vi "Simulation Configuration from Command-Line.vi"(8 "error in":errorcluster, 11 "simulation configuration in":T1={"maxTime"=5.0, "enableVisualization"=TRUE, "statechart"=path "iRobot Navigation State Machine.vi", "environment"=path "iRobot Navigation State Machine.vi", "record"=path "Simulation Record.xml", "autograde?"=TRUE, "interactive?"=FALSE, "feedback mode"=enum."debug navigation"}) -> (0 "error out":errorcluster, 3 "simulation configuration out":T1={"maxTime"=5.0, "enableVisualization"=TRUE, "statechart"=path "iRobot Navigation State Machine.vi", "environment"=path "iRobot Navigation State Machine.vi", "record"=path "Simulation Record.xml", "autograde?"=TRUE, "interactive?"=FALSE, "feedback mode"=enum."debug navigation"})   [LabVIEW 2013]
uses:
  CyberSim interface/Simulation Configuration.ctl
  autograder/feedbackMode.ctl
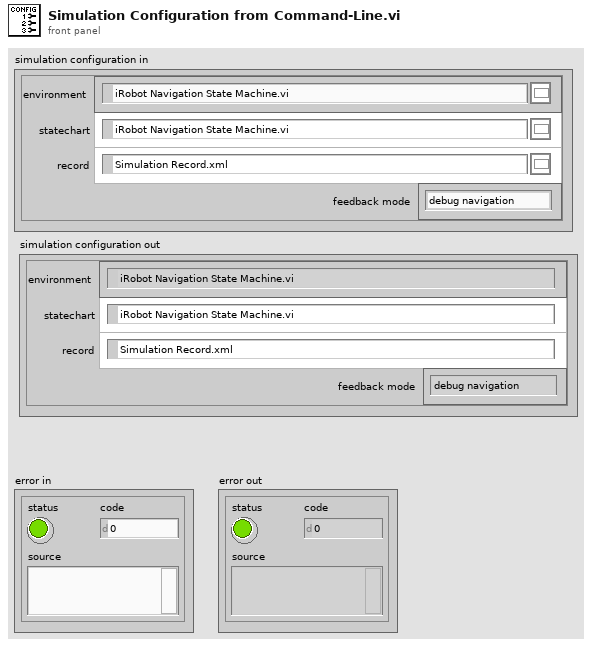
[diagram p1: front panel]
types:
  T1 = typedef "Simulation Configuration.ctl" = cluster{"maxTime":sgl, "enableVisualization":bool, "statechart":path, "environment":path, "record":path, "autograde?":bool, "interactive?":bool, "feedback mode":T2}
  T2 = typedef "feedbackMode.ctl" = enum32{"debug navigation", "debug hill climb", "autograde navigation", "autograde hill climb"}
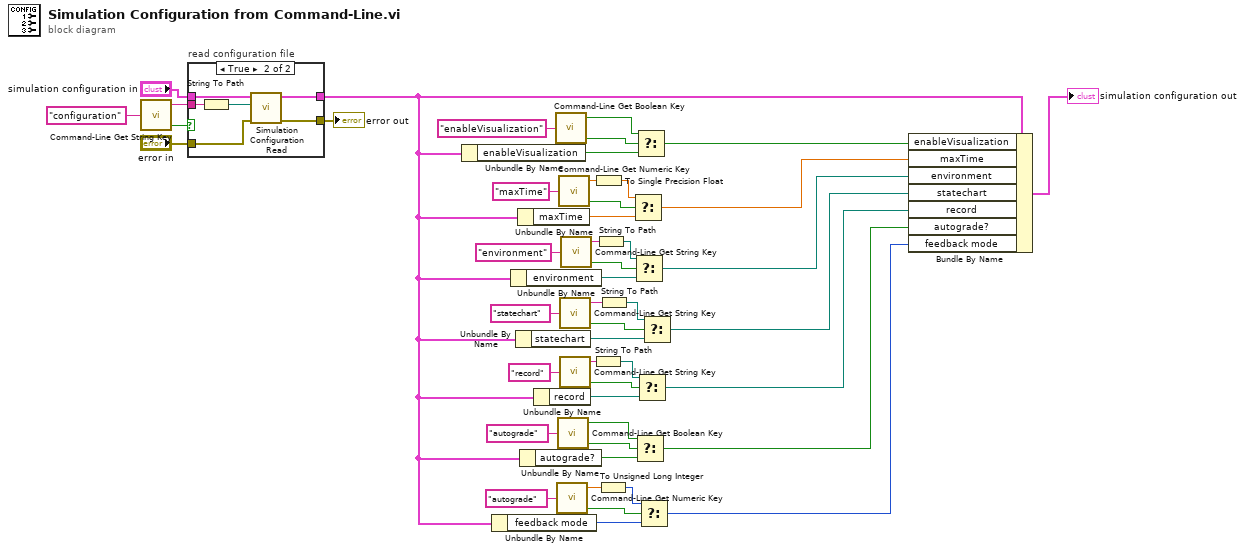
[diagram p0: block diagram]
diagram:
  n1 = call "Command-Line Get String Key.vi"("string key"="configuration") -> ("key found?"=w42:bool, "string value"=w41:string)  [unwired: 3 in]
  n2 = case "read configuration file" shown="True" w42 {
    tunnel: w41 -> [_ w56]
    tunnel: "simulation configuration in" -> [w50 w53]
    tunnel: [w50 w55] -> w4
    tunnel: "error in" -> [w49 w52]
    tunnel: [w49 w54] -> w13
    frame False {
    }
    frame True {
      n3 = String To Path(string=w56) -> (path=w51:path)
      n4 = call "Simulation Configuration Read.vi"("error in (no error)"=w52, "configuration"=w51, "simulation configuration"=w53) -> ("error out"=w54:errorcluster, "simulation configuration"=w55:T1)  [unwired: 7 in]
    }
  }
  "error out" <- w13
  n5 = Unbundle By Name(w4) -> ("enableVisualization"=w38:bool)
  n6 = Unbundle By Name(w4) -> ("feedback mode"=w5:T2)
  n7 = Unbundle By Name(w4) -> ("environment"=w34:path)
  n8 = Unbundle By Name(w4) -> ("statechart"=w19:path)
  n9 = Unbundle By Name(w4) -> ("maxTime"=w30:sgl)
  n10 = Unbundle By Name(w4) -> ("autograde?"=w10:bool)
  n11 = Unbundle By Name(w4) -> ("record"=w15:path)
  n12 = call "Command-Line Get Boolean Key.vi"("boolean key"="enableVisualization" ("string key")) -> ("key found?"=w37:bool, "boolean value"=w36:bool)  [unwired: 3 in]
  n13 = call "Command-Line Get Numeric Key.vi"("numeric key"="autograde") -> ("key found?"=w6:bool, "numeric value"=w3:dbl)  [unwired: 3 in]
  n14 = call "Command-Line Get Boolean Key.vi"("boolean key"="autograde" ("numeric key")) -> ("key found?"=w11:bool, "boolean value"=w9:bool)  [unwired: 3 in]
  n15 = call "Command-Line Get Numeric Key.vi"("numeric key"="maxTime") -> ("key found?"=w29:bool, "numeric value"=w28:dbl)  [unwired: 3 in]
  n16 = call "Command-Line Get String Key.vi"("string key"="statechart") -> ("key found?"=w20:bool, "string value"=w39:string)  [unwired: 3 in]
  n17 = call "Command-Line Get String Key.vi"("string key"="record" ("numeric key")) -> ("key found?"=w22:bool, "string value"=w35:string)  [unwired: 3 in]
  n18 = call "Command-Line Get String Key.vi"("string key"="environment" ("numeric key")) -> ("key found?"=w31:bool, "string value"=w33:string)  [unwired: 3 in]
  n19 = String To Path(string=w35) -> (path=w23:path)
  n20 = To Single Precision Float(number=w28) -> (single precision float=w27:sgl)
  n21 = String To Path(string=w33) -> (path=w32:path)
  n22 = To Unsigned Long Integer(number=w3) -> (unsigned 32bit integer=w2:u32)
  n23 = String To Path(string=w39) -> (path=w18:path)
  n24 = Select(t=w27, s=w29, f=w30) -> (s? t:f=w24:sgl)
  n25 = Select(t=w32, s=w31, f=w34) -> (s? t:f=w21:path)
  n26 = Select(t=w9, s=w11, f=w10) -> (s? t:f=w8:bool)
  n27 = Select(t=w36, s=w37, f=w38) -> (s? t:f=w26:bool)
  n28 = Select(t=w23, s=w22, f=w15) -> (s? t:f=w14:path)
  n29 = Select(t=w2, s=w6, f=w5) -> (s? t:f=w1:u32)
  n30 = Select(t=w18, s=w20, f=w19) -> (s? t:f=w17:path)
  n31 = Bundle By Name(cluster=w4, "enableVisualization"=w26, "maxTime"=w24, "environment"=w21, "statechart"=w17, "record"=w14, "autograde?"=w8, "feedback mode"=w1) -> (→"simulation configuration out":T1)
